vi "Update Record.vi"(8 "error in (no error)":errorcluster, 10 "Records":T1 {"Step Duration" format="%#_5f"}, 11 "Simulated Configuration Database Actor in":refnum<class "Sim Configuration Database Actor.lvclass">) -> (0 "error out":errorcluster, 3 "Simulated Configuration Database Actor out":refnum<class "Sim Configuration Database Actor.lvclass">)   [LabVIEW 2019, in "Sim Configuration Database Actor.lvlib" / "Sim Configuration Database Actor.lvclass"]
uses:
  Sim Configuration Database Actor.lvclass
  Records.ctl
  Sim Configuration Database Actor.lvclass/Sim Configuration Database Actor.ctl
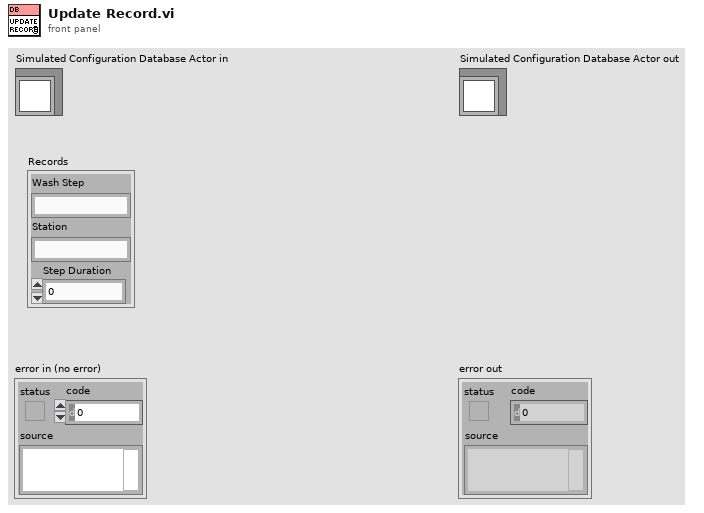
[diagram p1: front panel]
types:
  T1 = typedef "Sim Configuration Database Actor.lvlib/Sim Configuration Database Actor.lvclass/Records.ctl" = cluster{"Wash Step":string, "Station":string, "Step Duration":u32}
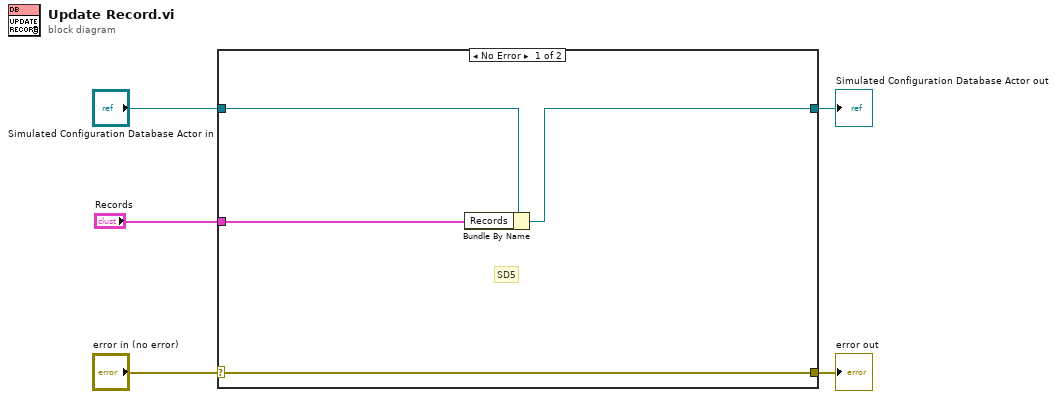
[diagram p0: block diagram]
diagram:
  n1 = case shown="No Error" "error in (no error)" {
    selector: "error in (no error)" -> [w9 w11]
    tunnel: [w9 w11] -> w4
    tunnel: [w6 w10] -> w2
    tunnel: "Simulated Configuration Database Actor in" -> [w8 w10]
    tunnel: "Records" -> [w7 _]
    frame No Error {
      # "SD5"
      n2 = Bundle By Name(cluster=w8, "Records"=w7) -> (w6:refnum<class "Sim Configuration Database Actor.lvclass">)
    }
    frame Error {
    }
  }
  "error out" <- w4
  "Simulated Configuration Database Actor out" <- w2
